vi "Get settings chain.vi"(8 "error in (no error)":errorcluster, 11 "Cascade512II Basein":refnum<class "DAQCascade512II.lvclass">) -> (0 "error out":errorcluster, 1 "class name":string[](array[string]), 2 "settings":variant[](array[variant]), 3 "Cascade512II Baseout":refnum<class "DAQCascade512II.lvclass">)   [LabVIEW 2012, in "DAQCascade512II.lvclass"]
doc: "Returns an array of variants containing the settings clusters of each class in the inheritance chain (lowest child class first), together with an array of all class names in the inheritance chain.\n\nFor classes without settings cluster, the settings chain contains empty variants."
uses:
  DAQCascade512II.lvclass
  <vilib>/Distrio/Murmex/Murmex/Murmex.lvclass
  DAQCascade512II.lvclass/DAQCascade512II.ctl
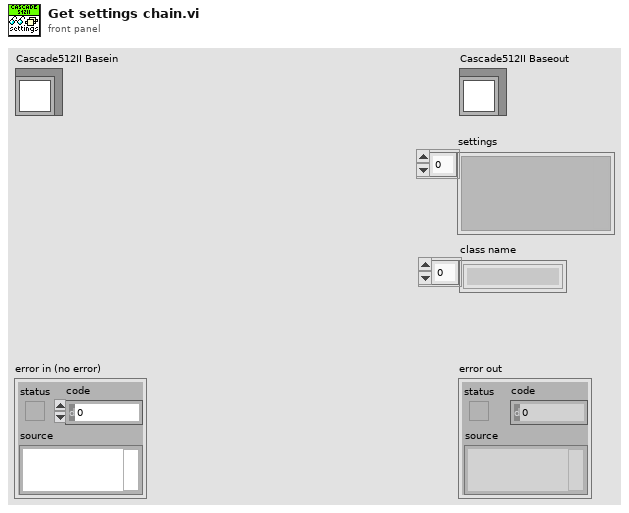
[diagram p1: front panel]
types:
  T1 = cluster{"Exposure (sec)":dbl, "number of frames":u32}
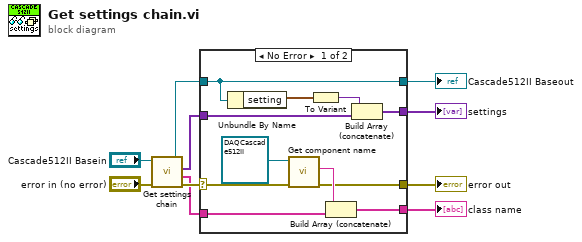
[diagram p0: block diagram]
diagram:
  n1 = call-parent "Get settings chain.vi"("error in (no error)"="error in (no error)", "MurmexBase in"="Cascade512II Basein") -> ("error out"=w4:errorcluster, "class name"=w2:string[], "settings"=w8:variant[], "MurmexBase out"=w6:refnum<class "DAQCascade512II.lvclass">)  [unwired: 6 in]
  n2 = case shown="No Error" w4 {
    selector: w4 -> [w16 w23]
    tunnel: w8 -> [w21 w24]
    tunnel: [w20 w24] -> w7
    tunnel: w6 -> [w14 w25]
    tunnel: [w14 w25] -> w5
    tunnel: [w15 w23] -> w3
    tunnel: w2 -> [w19 w22]
    tunnel: [w17 w22] -> w1
    frame No Error {
      n3 = Unbundle By Name(w14) -> ("setting"=w13:T1)
      n4 = call <vilib>:"Get component name.vi"("error in (no error)"=w16, "Murmex in"=refnum<class "DAQCascade512II.lvclass"> refnum ("DAQCascade512II")) -> ("error out"=w15:errorcluster, "component name"=w18:string)  [unwired: 7 in, 1 out]
      n5 = To Variant(anything=w13) -> (Variant=w12:variant)
      n6 = Build Array (concatenate)(w18, w19) -> (w17:string[])
      n7 = Build Array (concatenate)(w12, w21) -> (w20:variant[])
    }
    frame Error {
    }
  }
  "error out" <- w3
  "Cascade512II Baseout" <- w5
  "settings" <- w7
  "class name" <- w1
